vi "VCS Set Protocol Stack Settings.vi"(8 "error in (no error)":errorcluster, 10 "settings":cluster{"baudrate":u32, "timeout":u32}, 11 "keyHandle in":u32) -> (0 "error out":errorcluster, 3 "keyHandle out":u32)   [LabVIEW 2018]
doc: "<B>VCS Set Protocol Stack Settings</B> writes the communication parameters. For exact values of baudrate use the function <B>VCS Get Baudrate Selection</B>."
uses:
  Resources/EposCmd.dll
  Resources/EposCmd64.dll
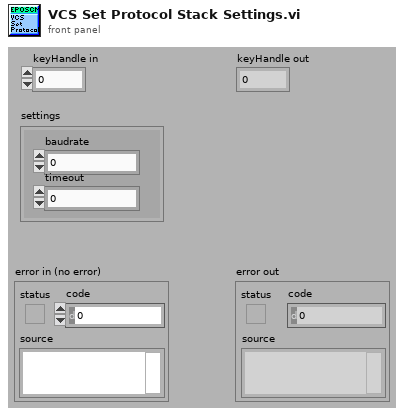
[diagram p1: front panel]
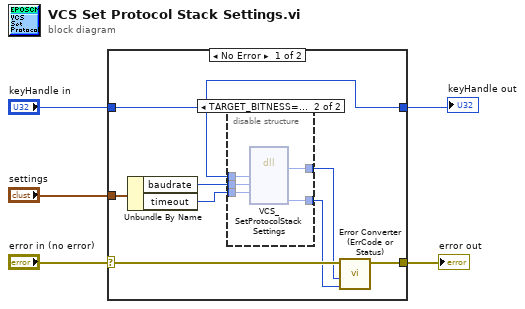
[diagram p0: block diagram]
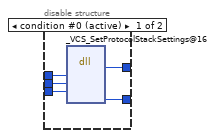
[diagram p2: hidden frame]
diagram:
  n1 = case shown="No Error" "error in (no error)" {
    selector: "error in (no error)" -> [w13 w25]
    tunnel: [w12 w25] -> w4
    tunnel: "settings" -> [w10 _]
    tunnel: "keyHandle in" -> [w7 w24]
    tunnel: [w7 w24] -> w1
    frame No Error {
      n2 = Unbundle By Name(w10) -> ("baudrate"=w9:u32, "timeout"=w8:u32)
      n3 = disable-structure shown="TARGET_BITNESS==64" {
        disable-tunnel: [w18 w23] -> w11
        disable-tunnel: w9 -> [w17 w22]
        disable-tunnel: w8 -> [w16 w21]
        disable-tunnel: w7 -> [w15 w20]
        disable-tunnel: [w14 w19] -> w6
        frame condition #0 (active) {
          n4 = dll-call lib="C:/Projeto em LabVIEW/EPOS-LabVIEW-Instrument-Driver-En/LabVIEW/maxon EPOS/Resources/EposCmd.*" fn="_VCS_SetProtocolStackSettings@16"("KeyHandle"=w15, "Baudrate"=w17, "Timeout"=w16) -> (w14:i32, "pErrorCode"=w18:u32)  [unwired: 7 in, 2 out]
        }
        frame condition #1 {
          n5 = dll-call lib="C:/setup/Resources/EposCmd64.dll" fn="VCS_SetProtocolStackSettings" ("EposCmd.dll:_VCS_SetProtocolStackSettings@16")("KeyHandle"=w20, "Baudrate"=w22, "Timeout"=w21) -> ("return type"=w19:i32, "pErrorCode"=w23:u32)  [unwired: 7 in, 2 out]
        }
      }
      n6 = call "Error Converter (ErrCode or Status).vi"("error code"=w11, "return type"=w6, "error in (no error)"=w13) -> ("error out"=w12:errorcluster)  [unwired: 7 in]
    }
    frame Error {
    }
  }
  "error out" <- w4
  "keyHandle out" <- w1
